vi "Configure Correction Frequency.vi"(8 "error in (no error)":errorcluster, 9 "Correction Frequency (50.0 MHz )":dbl=50000000.0 min=1000.0 max=1000000000000.0 format="%#.6g", 11 "VISA resource name":refnum<visa-resource-name>) -> (0 "error out":errorcluster, 3 "VISA resource name out":refnum<visa-resource-name>)   [LabVIEW 2011, in "Template - Power Meter.lvlib"]
doc: "Configure the Correction Frequency settings which will assist the instrument in making an accurate measurement."
uses:
  <instrlib>/_Template - Power Meter/Template - Power Meter.lvlib
panel:
  in  "Channel (1: Channel A)":u16(ring)=1 items=["Channel A"=1, "Channel B"=2]
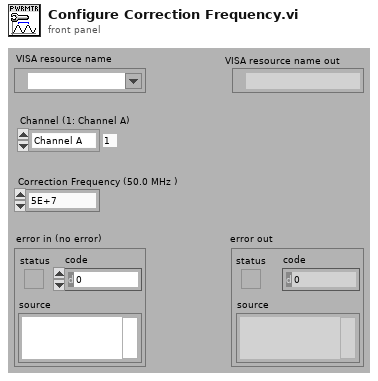
[diagram p1: front panel]
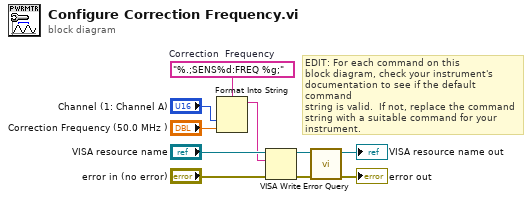
[diagram p0: block diagram]
diagram:
  w4 = "%.;SENS%d:FREQ %g;"  # Correction  Frequency
  # "EDIT: For each command on this\nblock diagram, check your instrument's\ndocumentation to see if the default command\nstring is valid.  If not, replace the command\nstring with a suitable command for your\ninstrument."
  n1 = Format Into String(format string=w4, "Channel (1: Channel A)", "Correction Frequency (50.0 MHz )") -> (resulting string=w2:string)  [unwired: 2 in, 1 out]
  n2 = VISA Write(VISA resource name="VISA resource name", write buffer=w2, error in (no error)="error in (no error)") -> (VISA resource name out=w8:refnum<visa-resource-name>, error out=w6:errorcluster)  [unwired: 1 out]
  n3 = call <instrlib>:"Error Query.vi"("error in (no error)"=w6, "VISA resource name"=w8) -> ("error out"=→"error out":errorcluster, "VISA resource name out"=→"VISA resource name out":refnum<visa-resource-name>)  [unwired: 6 in, 2 out]
